vi "Error Cluster to Array of Errors.vi"(11 "error":errorcluster) -> (3 "array of errors":errorcluster[](array[cluster]))   [LabVIEW 2020, in "Multi Error Cluster.lvlib"]
doc: "Converts a cluster of errors into an array of encoded errors. This VI returns an empty array if the error cluster does not include any errors."
uses:
  <vilib>/MultiError/TokenizeJSON/Multi Error Cluster.lvlib
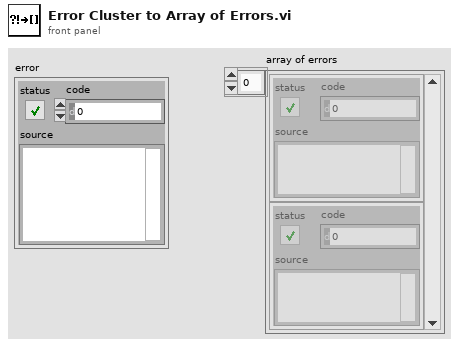
[diagram p1: front panel]
types:
  T1 = typedef "Multi Error Cluster.lvlib/JSON Token Descriptor.ctl" = cluster{"match string":string, "raw token type":T2, "byte offset ":i32}
  T2 = typedef "Multi Error Cluster.lvlib/JSON Raw Token Values.ctl" = enum32{"{", "}", "[", "]", ",", ":", "\"", "number", "string", "true", "false", "null", "invalid"}
  T3 = typedef "Multi Error Cluster.lvlib/JSON Token Values.ctl" = enum32{"array begin", "array end", "object begin", "object end", "value", "invalid", "name"}
  T4 = typedef "Multi Error Cluster.lvlib/JSON Object Descriptor.ctl" = cluster{"begin info":T1, "end info":T1, "begin Index":i32, "end Index":i32}
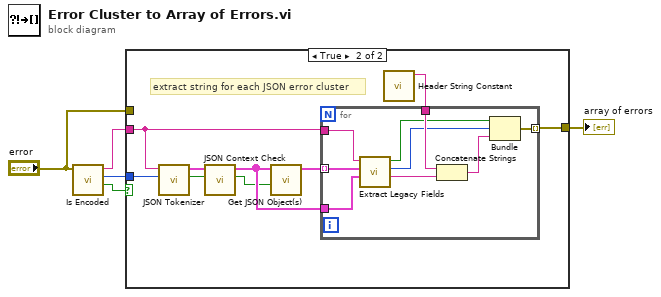
[diagram p0: block diagram]
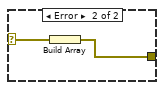
[diagram p3: hidden frame]
diagram:
  n1 = call <vilib>:"Is Encoded.vi"("error in (no error)"="error") -> ("Is Encoded"=w4:bool, "offset past"=w3:i32, "source"=w2:string)  [unwired: 8 in]
  n2 = case shown="True" w4 {
    tunnel: [w7 w17] -> w5
    tunnel: w2 -> [_ w11]
    tunnel: "error" -> [w6 _]
    tunnel: w3 -> [_ w10]
    frame False {
      # "Legacy error"
      n3 = case shown="No Error" w6 {
        selector: w6 -> [_ w8]
        tunnel: [_ w9] -> w7
        frame No Error {
        }
        frame Error {
          n4 = Build Array(w8) -> (w9:errorcluster[])
        }
      }
    }
    frame True {
      # "extract string for each JSON error cluster"
      n5 = call <vilib>:"JSON Tokenizer.vi"("string offset"=w10, "JSON String"=w11) -> ("Invalid"=w15:bool, "Array"=w14:T1[])  [unwired: 8 in]
      n6 = call <vilib>:"JSON Context Check.vi"("Invalid in"=w15, "Parse Tokens in"=w14) -> ("Invalid out"=w13:bool, "tokens"=w16:cluster{"token type":T3, T1}[])  [unwired: 8 in]
      n7 = call <vilib>:"Get JSON Object(s).vi"("invalid in"=w13, "tokens"=w16) -> ("array of JSON objects"=w18:T4[])  [unwired: 9 in]
      n8 = call <vilib>:"Header String Constant.vi"() -> ("Single Header String"=w12:string)  [unwired: 10 in, 1 out]
      n9 = for {
        tunnel: w18 -> [w27] mode=indexing
        tunnel: w11 -> [w26]
        tunnel: [w25] -> w17 mode=indexing
        tunnel: w16 -> [w24]
        tunnel: w12 -> [w22]
        n10 = call <vilib>:"Extract Legacy Fields.vi"("Checked Tokens in"=w24, "JSON Object Descriptor"=w27, "source in"=w26) -> ("source out"=w21:string, "code"=w20:i32, "status"=w19:bool)  [unwired: 6 in]
        n11 = Concatenate Strings(w22, w21) -> (w23:string)
        n12 = Bundle("status"=w19, "code"=w20, w23) -> (w25:cluster{"status":bool, "code":i32, string})  [unwired: 1 in]
      }
    }
  }
  "array of errors" <- w5
